vi "instance count allowed.vi"(8 "error in":errorcluster, 11 "Profibus Module configuration in":refnum<class "Profibus Module configuration.lvclass">) -> (0 "error out":errorcluster, 2 "instances allowed":i32, 3 "Profibus Module configuration out":refnum<class "Profibus Module configuration.lvclass">)   [LabVIEW 2013, in "Profibus Module configuration.lvclass"]
uses:
  Profibus Module configuration.lvclass
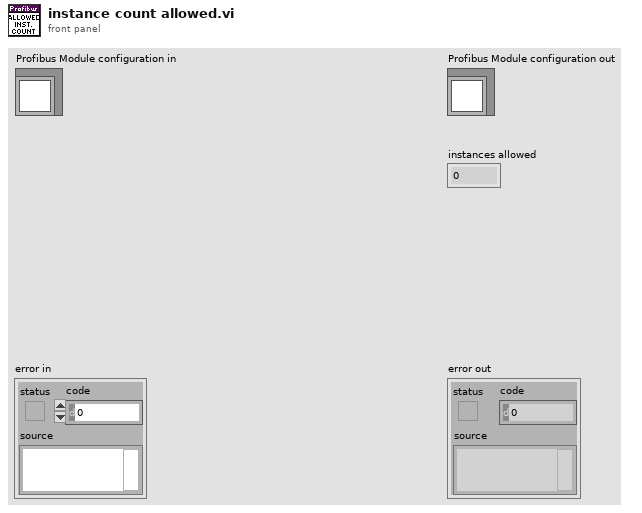
[diagram p1: front panel]
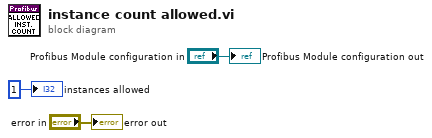
[diagram p0: block diagram]
diagram:
  "error out" <- "error in"
  "Profibus Module configuration out" <- "Profibus Module configuration in"
  "instances allowed" <- 1 ("instances allowed")
